vi "writeToXML.vi"(8 "error in (no error)":errorcluster, 10 "Class Label":string="RotatorTracking", 11 "RotatorTracking in":refnum<class "RotatorTracking.lvclass">) -> (0 "error out":errorcluster, 2 "XML out":string="<RotatorTracking>\n  <cableWrapDesired>C</cableWrapDesired>\n  <np>0</np>\n  <rotVelocity>0</rotVelocity>\n  <time>0</time>\n</RotatorTracking>", 3 "RotatorTracking out":refnum<class "RotatorTracking.lvclass">)   [LabVIEW 2014, in "TCSDataDefinitions.lvlib" / "TCSMountControlStatus.lvlib" / "RotatorTracking.lvclass"]
uses:
  RotatorTracking.lvclass
  <userlib>/Common/UnitsAndXML/FlattenItemWithUnitToXML/FlattenPlaneAngleToXML/PlaneAngleUnit.ctl
  <userlib>/Common/UnitsAndXML/FlattenItemWithUnitToXML/FlattenAngularVelocityToXML/AngularVelocityUnit.ctl
  <userlib>/Common/UnitsAndXML/FlattenItemWithUnitToXML/FlattenTimeToXML/TimeUnit.ctl
  RotatorTracking.lvclass/RotatorTracking.ctl
  <userlib>/Common/UnitsAndXML/UnitsAndXML.lvlib
  <userlib>/Common/XML/XMLGenerator/XMLGenerator.lvclass
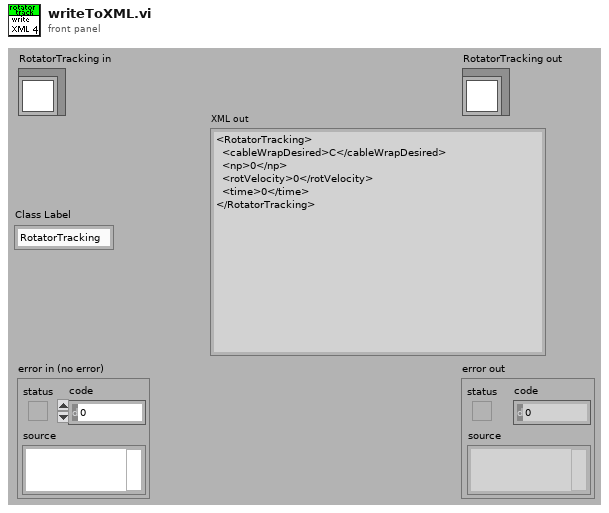
[diagram p1: front panel]
types:
  T1 = typedef "UnitsAndXML.lvlib/TimeUnit.ctl" = enum16{"s", "d", "h", "min", "a"}
  T2 = typedef "UnitsAndXML.lvlib/AngularVelocityUnit.ctl" = enum16{"\"/a", "deg/s", "\"/s"}
  T3 = typedef "UnitsAndXML.lvlib/PlaneAngleUnit.ctl" = enum16{"rad", "deg", "'", "\""}
  T4 = typedef "TCSDataDefinitions.lvlib/TCSMountControlStatus.lvlib/CableWrapDesired.ctl" = enum16{"C", "W", "S"}
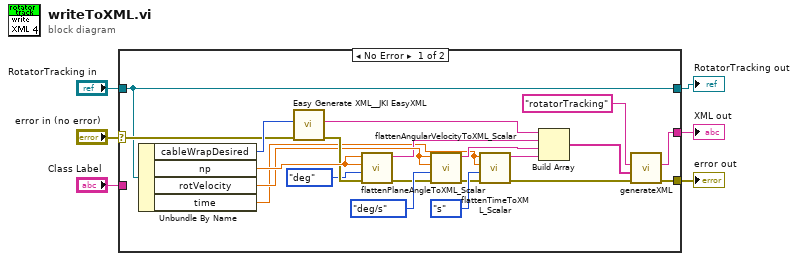
[diagram p0: block diagram]
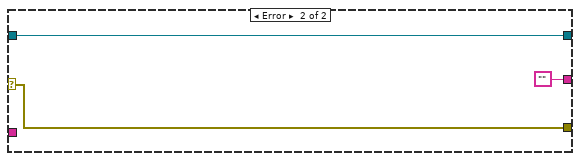
[diagram p2: hidden frame]
diagram:
  n1 = case shown="No Error" "error in (no error)" {
    selector: "error in (no error)" -> [w26 w30]
    tunnel: [w25 w30] -> w5
    tunnel: [w8 w29] -> w3
    tunnel: "RotatorTracking in" -> [w8 w29]
    tunnel: [w22 ""] -> w2
    tunnel: "Class Label" -> [_ _]
    frame No Error {
      n2 = Unbundle By Name(w8) -> ("cableWrapDesired"=w27:T4, "np"=w21:dbl[unit], "rotVelocity"=w18:dbl[unit], "time"=w13:dbl[unit])
      n3 = call <vilib>:"Easy Generate XML__JKI EasyXML.vi"("error in (no error)"=w26, "LabVIEW Data"=w27) -> ("error out"=w20:errorcluster, "XML String"=w24:string)  [unwired: 8 in]
      n4 = call <userlib>:"flattenPlaneAngleToXML_Scalar.vi"("error in (no error)"=w20, "planeAngleUnitInXML"=PlaneAngleUnit."deg", "planeAngleAgain"=w21, "planeAngle"=w21) -> ("error out"=w16:errorcluster, "xmlString"=w15:string)  [unwired: 6 in]
      n5 = call <userlib>:"flattenAngularVelocityToXML_Scalar.vi"("error in (no error)"=w16, "angularVelocityUnitInXML"=AngularVelocityUnit."deg/s", "anuglarVelocityAgain"=w18, "angularVelocity"=w18) -> ("error out"=w11:errorcluster, "xmlString"=w14:string)  [unwired: 6 in]
      n6 = call <userlib>:"flattenTimeToXML_Scalar.vi"("error in (no error)"=w11, "timeUnitInXML"=TimeUnit."s", "timeAgain"=w13, "time"=w13) -> ("error out"=w10:errorcluster, "xmlString"=w9:string)  [unwired: 6 in]
      n7 = Build Array(w24, w15, w14, w9) -> (w23:string[])
      n8 = call <userlib>:"generateXML.vi"("error in"=w10, "childrenXML"=w23, "elementName"="rotatorTracking" ("Class Label")) -> ("error out"=w25:errorcluster, "XML out"=w22:string)  [unwired: 6 in, 1 out]
    }
    frame Error {
    }
  }
  "error out" <- w5
  "RotatorTracking out" <- w3
  "XML out" <- w2
